vi "Container.vi"(10 "SubPnl Refnum":refnum<vi>, 11 "Notifier":refnum<notifier>) -> ()   [LabVIEW 2013, in "main.lvlib"]
uses:
  main.lvlib
panel:
  out "Waveform Chart":dbl(graph)
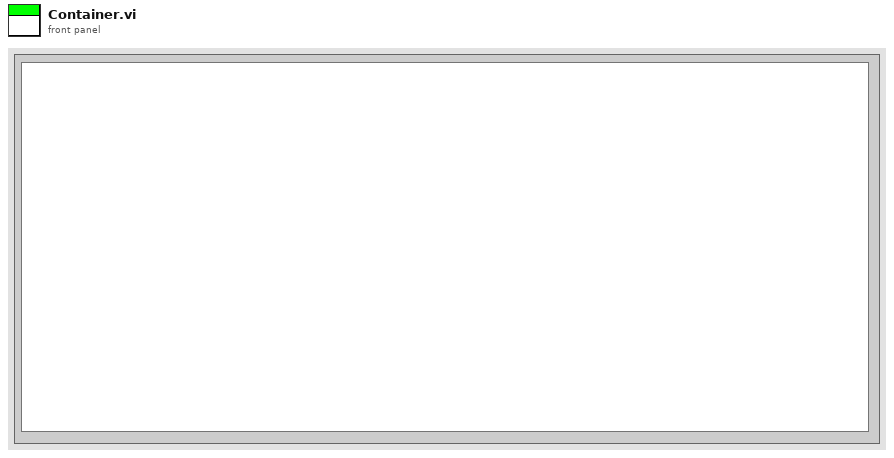
[diagram p1: front panel]
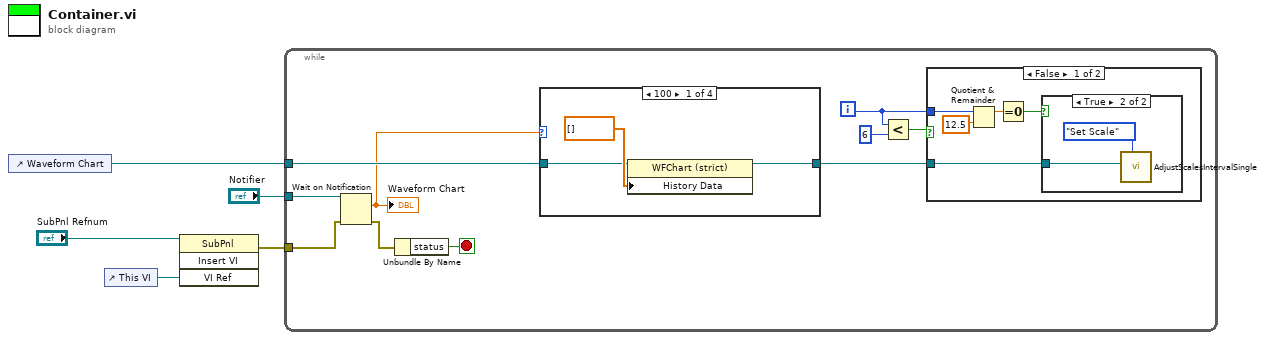
[diagram p0: block diagram]
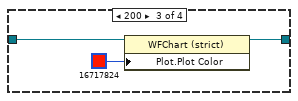
[diagram p3: hidden frame]
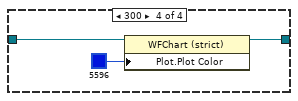
[diagram p4: hidden frame]
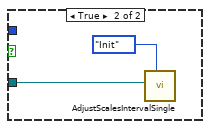
[diagram p6: hidden frame]
diagram:
  n1 = control-ref of="Waveform Chart"() -> (w1:refnum<vi>)
  n2 = control-ref of="This VI"() -> (w3:refnum<vi>)
  n3 = invoke class="SubPnl" method="Insert VI"(reference="SubPnl Refnum", "VI Ref"=w3) -> (error out=w2:errorcluster)  [unwired: 2 in, 3 out]
  n4 = while {
    tunnel: "Notifier" -> [w15]
    tunnel: w2 -> [w12]
    tunnel: w1 -> [w8]
    i -> [w11]
    stop <- w13 stop-if-true
    n5 = Wait on Notification(notifier=w15, error in (no error)=w12) -> (notification=w7:dbl, error out=w14:errorcluster)  [unwired: 2 in, 2 out]
    "Waveform Chart" <- w7
    n6 = Unbundle By Name(w14) -> ("status"=w13:bool)
    n7 = case shown="100" w7 {
      tunnel: w8 -> [w17 w19 w21 w24]
      tunnel: [w16 w19 w20 w23] -> w6
      frame 100 {
        n8 = property class="WFChart (strict)"(reference=w17, "History Data"=dbl[] []) -> (reference out=w16:refnum<vi>)  [unwired: 1 in, 1 out]
      }
      frame Default {
      }
      frame 200 {
        n9 = property class="WFChart (strict)"(reference=w21, "Plot.Plot Color"=u32 16717824) -> (reference out=w20:refnum<vi>)  [unwired: 1 in, 1 out]
      }
      frame 300 {
        n10 = property class="WFChart (strict)"(reference=w24, "Plot.Plot Color"=u32 5596) -> (reference out=w23:refnum<vi>)  [unwired: 1 in, 1 out]
      }
    }
    n11 = Less?(x=w11, y=6) -> (x < y?=w9:bool)
    n12 = case shown="False" w9 {
      tunnel: w6 -> [w30 w33]
      tunnel: w11 -> [w26 _]
      frame False {
        n13 = Quotient & Remainder(x=w26, y=12.5) -> (x-y*floor(x/y)=w28:dbl)  [unwired: 1 out]
        n14 = Equal To 0?(x=w28) -> (x = 0?=w27:bool)
        n15 = case shown="True" w27 {
          tunnel: w30 -> [_ w32]
          frame False {
          }
          frame True {
            n16 = call "AdjustScalesIntervalSingle.vi"("Action"=enum16{"Init", "Set Scale"}."Set Scale", "WFChart Refnum"=w32) -> ()  [unwired: 10 in]
          }
        }
      }
      frame True {
        n17 = call "AdjustScalesIntervalSingle.vi"("Action"=enum16{"Init", "Set Scale"}."Init", "WFChart Refnum"=w33) -> ()  [unwired: 10 in]
      }
    }
  }
